vi "Read and Check Faults.vi"(6 "DMMVoltageFaultUpperLimit":dbl, 8 "error in (no error)":errorcluster, 9 "SMUSequenceNumberOfSteps":i32, 10 "DMM Ref":refnum<k15>, 11 "SMU Ref":refnum<k15>) -> (0 "error out":errorcluster, 1 "Result":T1, 2 "DMM Ref Out":refnum<k15>, 3 "SMU Ref Out":refnum<k15>)   [LabVIEW 2019]
uses:
  Result.ctl
  ErrorOutData.ctl
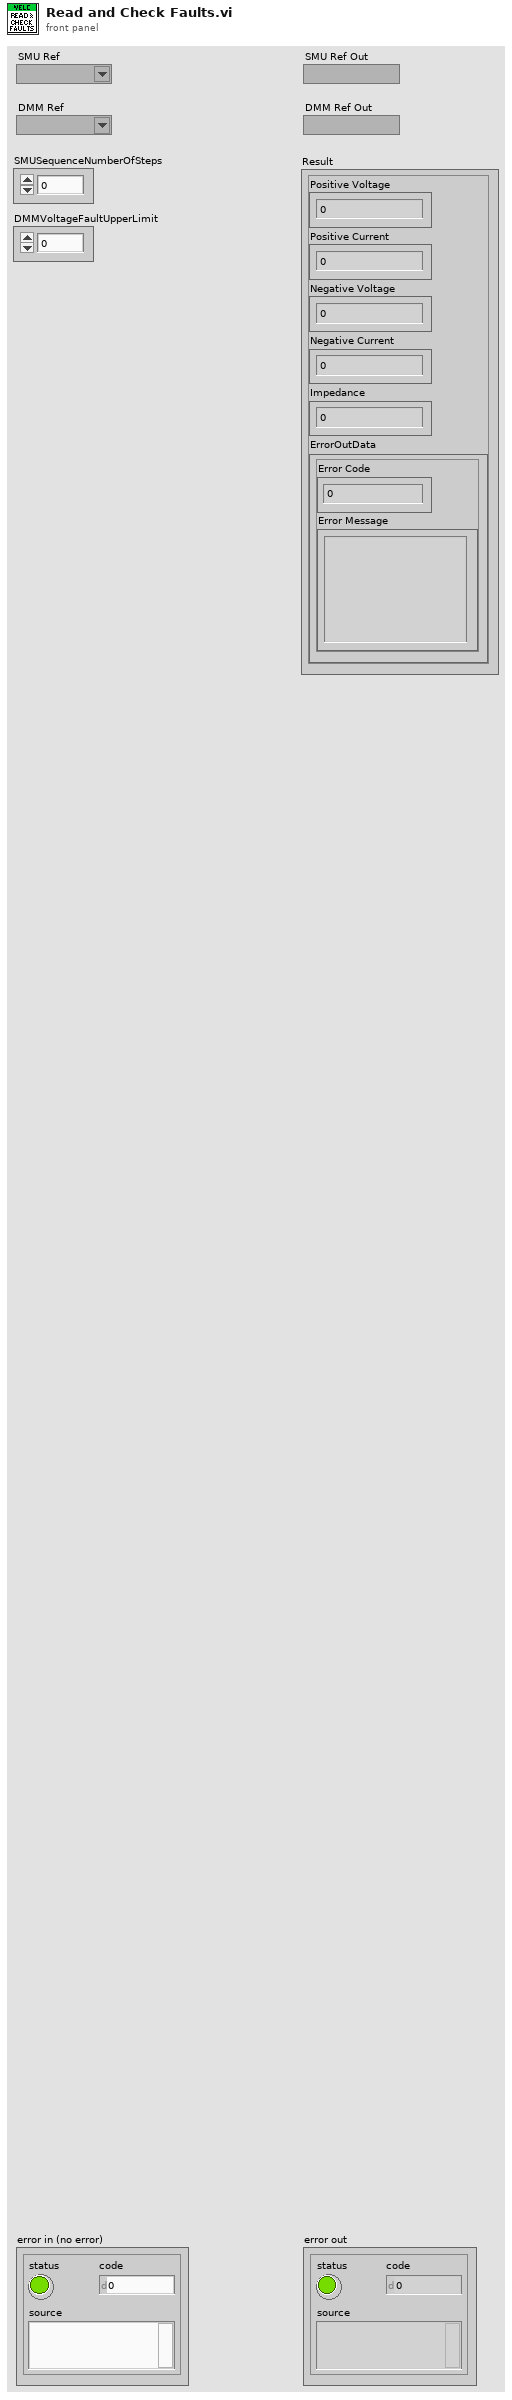
[diagram p1: front panel]
types:
  T1 = typedef "Result.ctl" = cluster{"Positive Voltage":dbl, "Positive Current":dbl, "Negative Voltage":dbl, "Negative Current":dbl, "Impedance":dbl, "ErrorOutData":T2}
  T2 = typedef "ErrorOutData.ctl" = cluster{"Error Code":i32, "Error Message":string}
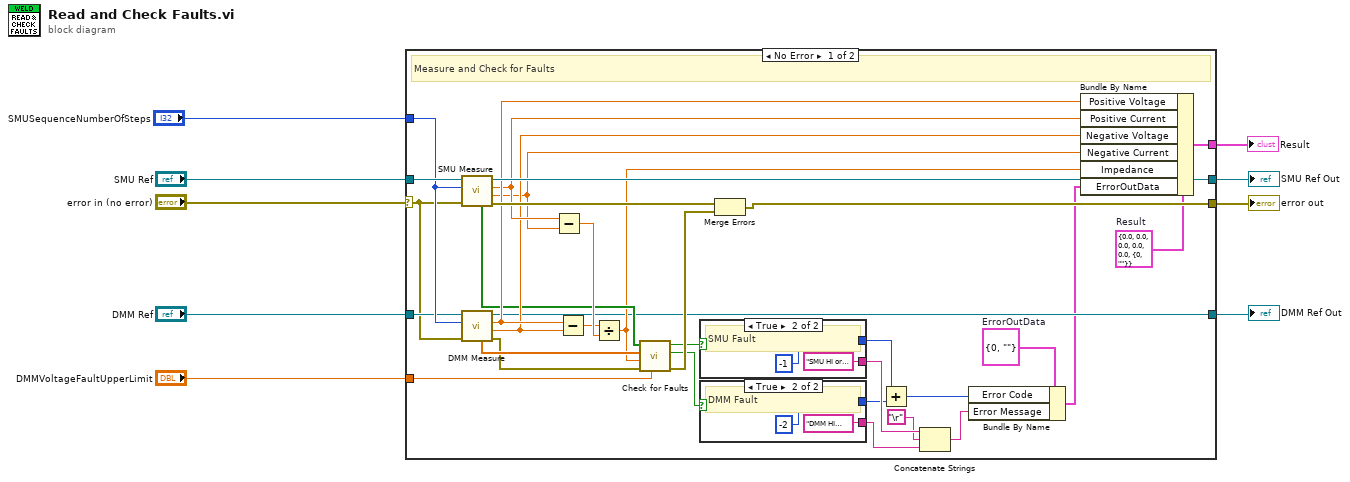
[diagram p0: block diagram]
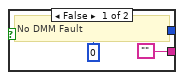
[diagram p2: hidden frame]
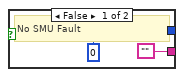
[diagram p3: hidden frame]
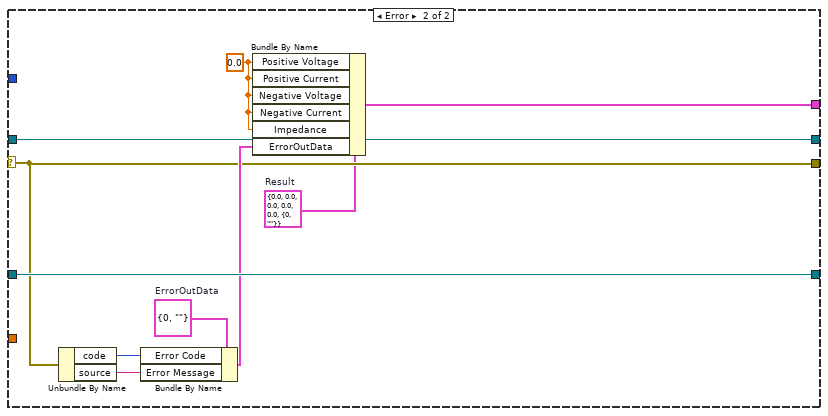
[diagram p4: hidden frame]
diagram:
  n1 = case shown="No Error" "error in (no error)" {
    selector: "error in (no error)" -> [w15 w54]
    tunnel: [w42 w60] -> w4
    tunnel: [w10 w55] -> w1
    tunnel: "SMU Ref" -> [w21 w60]
    tunnel: "SMUSequenceNumberOfSteps" -> [w20 _]
    tunnel: "DMM Ref" -> [w19 w59]
    tunnel: [w17 w59] -> w5
    tunnel: "DMMVoltageFaultUpperLimit" -> [w16 _]
    tunnel: [w14 w54] -> w6
    frame No Error {
      w12 = T1 {"Positive Voltage"=0.0, "Positive Current"=0.0, "Negative Voltage"=0.0, "Negative Current"=0.0, "Impedance"=0.0, "ErrorOutData"={"Error Code"=0, "Error Message"=""}}  # Result
      w13 = T2 {"Error Code"=0, "Error Message"=""}  # ErrorOutData
      # "Measure and Check for Faults"
      n2 = call "SMU Measure.vi"("error in (no error)"=w15, "SMUSequenceNumberOfSteps"=w20, "IVI Refnum in"=w21) -> ("error out"=w41:errorcluster, "Numeric"=w34:dbl, "Numeric 2"=w36:dbl, "IVI Refnum out"=w42:refnum<k15>, "in compliance"=w24:bool[])  [unwired: 4 in]
      n3 = call "DMM Measure.vi"("error in (no error)"=w15, "SMUSequenceNumberOfSteps"=w20, "IVI Refnum in"=w19) -> ("error out"=w18:errorcluster, "Numeric"=w35:dbl, "Numeric 2"=w37:dbl, "IVI Refnum out"=w17:refnum<k15>, "Measurements"=w23:dbl[])  [unwired: 4 in]
      n4 = Subtract(x=w36, y=w34) -> (x-y=w39:dbl)
      n5 = Subtract(x=w37, y=w35) -> (x-y=w38:dbl)
      n6 = Divide(x=w38, y=w39) -> (x/y=w22:dbl)
      n7 = call "Check for Faults.vi"("DMM Voltage Fault Upper Limit"=w16, "Error In"=w18, "Resistance In"=w22, "dmm voltage measurements"=w23, "in compliance"=w24) -> ("Error Out"=w40:errorcluster, "DMM Fault"=w28:bool, "SMU Fault"=w32:bool)  [unwired: 3 in, 1 out]
      n8 = case shown="True" w32 {
        tunnel: ["" "SMU HI or LO lead disconnected\n- SMU in compliance\n- SMU Fault = True"] -> w31
        tunnel: [0 -1] -> w29
        frame False {
          # "No SMU Fault"
        }
        frame True {
          # "SMU Fault"
        }
      }
      n9 = case shown="True" w28 {
        tunnel: ["" "DMM HI SENSE or LO SENSE lead disconnected\n- DMM measures NaN, or \n- DMM overrange warning, or\n- DMM voltage > DMM Voltage Fault Upper Limit "] -> w26
        tunnel: [0 -2] -> w25
        frame False {
          # "No DMM Fault"
        }
        frame True {
          # "DMM Fault"
        }
      }
      n10 = Merge Errors(w41, w40) -> (w14:errorcluster)
      n11 = Add(x=w29, y=w25) -> (x+y=w33:i32)
      n12 = Concatenate Strings(w31, "\r", w26) -> (w30:string)
      n13 = Bundle By Name(cluster=w13, "Error Code"=w33, "Error Message"=w30) -> (w11:T2)
      n14 = Bundle By Name(cluster=w12, "Positive Voltage"=w37, "Positive Current"=w36, "Negative Voltage"=w35, "Negative Current"=w34, "Impedance"=w22, "ErrorOutData"=w11) -> (w10:T1)
    }
    frame Error {
      w51 = T1 {"Positive Voltage"=0.0, "Positive Current"=0.0, "Negative Voltage"=0.0, "Negative Current"=0.0, "Impedance"=0.0, "ErrorOutData"={"Error Code"=0, "Error Message"=""}}  # Result
      w52 = T2 {"Error Code"=0, "Error Message"=""}  # ErrorOutData
      w53 = 0.0 ("Positive Voltage")
      n15 = Unbundle By Name(w54) -> ("code"=w56:i32, "source"=w57:string)
      n16 = Bundle By Name(cluster=w52, "Error Code"=w56, "Error Message"=w57) -> (w58:T2)
      n17 = Bundle By Name(cluster=w51, "Positive Voltage"=w53, "Positive Current"=w53, "Negative Voltage"=w53, "Negative Current"=w53, "Impedance"=w53, "ErrorOutData"=w58) -> (w55:T1)
    }
  }
  "error out" <- w6
  "DMM Ref Out" <- w5
  "SMU Ref Out" <- w4
  "Result" <- w1
